vi "Debounce.vi"(5 "Input":bool) -> (2 "Output":bool)   [LabVIEW 2017]
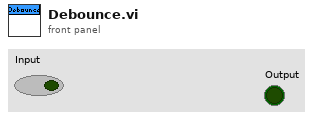
[diagram p1: front panel]
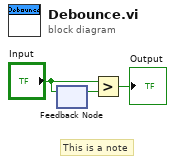
[diagram p0: block diagram]
diagram:
  # "This is a note"
  n1 = feedback-in #1("Input") -> ()
  n2 = feedback #1() -> (w2:bool)  [unwired: 1 in]
  n3 = Greater?(x="Input", y=w2) -> (0:→"Output":bool)
